vi "Error - StoreError.vi"(7 "Init?":bool, 8 "Error In":errorcluster, 11 "Error Source In":string) -> (0 "Error Out":errorcluster, 3 "Error Sources Out":string[](array[string]))   [LabVIEW 2011]
doc: "This Functional Global will store Error cluster if error has occured."
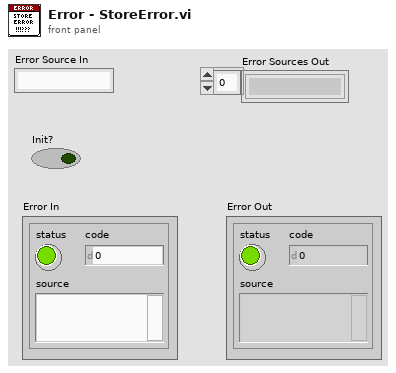
[diagram p1: front panel]
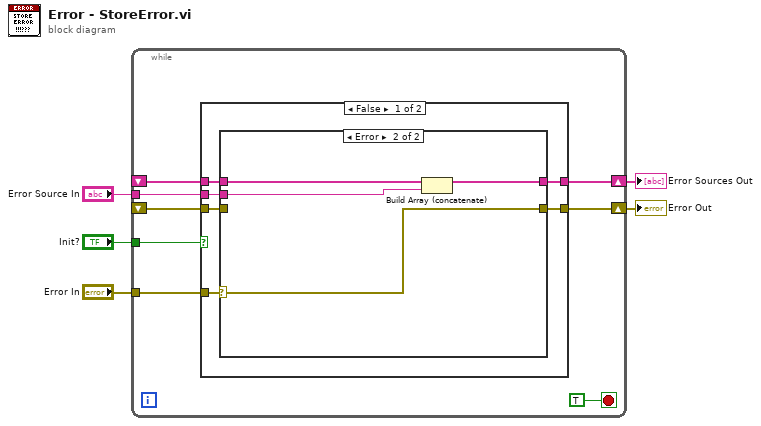
[diagram p0: block diagram]
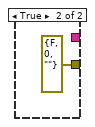
[diagram p3: hidden frame]
diagram:
  n1 = while {
    tunnel: "Error In" -> [w12]
    shift-right: [w11] -> w4
    shift-left: _ -> [w10]
    tunnel: "Init?" -> [w9]
    tunnel: "Error Source In" -> [w8]
    shift-right: [w7] -> w1
    shift-left: _ -> [w6]
    stop <- TRUE stop-if-true
    n2 = case shown="False" w9 {
      tunnel: w12 -> [w19 _]
      tunnel: [w18 errorcluster {"status"=FALSE, "code"=0, "source"=""} ("error IO")] -> w11
      tunnel: w10 -> [w17 _]
      tunnel: w8 -> [w16 _]
      tunnel: [w15 _] -> w7
      tunnel: w6 -> [w14 _]
      frame False {
        n3 = case shown="Error" w19 {
          selector: w19 -> [_ w25]
          tunnel: [w21 w25] -> w18
          tunnel: w17 -> [w21 _]
          tunnel: w16 -> [_ w24]
          tunnel: [w20 w23] -> w15
          tunnel: w14 -> [w20 w22]
          frame No Error {
          }
          frame Error {
            n4 = Build Array (concatenate)(w22, w24) -> (w23:string[])
          }
        }
      }
      frame True {
      }
    }
  }
  "Error Out" <- w4
  "Error Sources Out" <- w1
